vi "search_dir.vi"() -> ()   [LabVIEW 2019]
panel:
  in  "file_name":string
  in  "dir_path":path
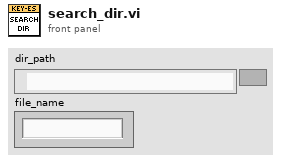
[diagram p1: front panel]
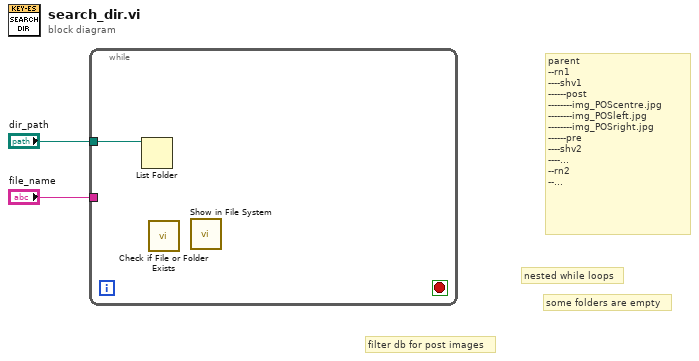
[diagram p0: block diagram]
diagram:
  # "filter db for post images"
  # "some folders are empty"
  # "nested while loops"
  # "parent\n--rn1\n----shv1\n------post\n--------img_POScentre.jpg\n--------img_POSleft.jpg\n--------img_POSright.jpg\n------pre\n----shv2\n----...\n--rn2\n--..."
  n1 = while {
    tunnel: "dir_path" -> [w3]
    tunnel: "file_name" -> [_]
    stop <- _ stop-if-true
    n2 = List Folder(path=w3) -> ()  [unwired: 3 in, 4 out]
    n3 = call <vilib>:"Check if File or Folder Exists.vi"() -> ()  [unwired: 9 in, 3 out]
    n4 = call <vilib>:"Show in File System.vi"() -> ()  [unwired: 11 in, 1 out]
  }
